vi "I2C_HostHandleIRQ_2.vi"(8 "error in":errorcluster, 10 "IRQ Number":i32, 11 "FPGA VI Reference In":T1) -> (0 "error out":errorcluster, 2 "Status":i16, 3 "FPGA VI Reference Out":T1)   [LabVIEW 2019]
doc: "Waits for the FPGA to update the specified IRQ. Once received it is acknowledged and the status is returned from the FPGA.\n\nVI Written By:\nPeter Fuller\nSenior Engineer\nplf Consulting, LLC"
uses:
  <vilib>/rvi/interface/nirviMethod/nirviMethod.xnode
  <vilib>/rvi/interface/nirviReadWriteControl/nirviReadWriteControl.xnode
  Controls/FPGA_Reference.ctl
  FPGA Bitfiles/LS_Durability_FPGA_9627.lvbitx
  <vilib>/rvi/interface/nirviMethod/StockFPGA_InlinedMethodWaitForSingleIRQ.vi
  <vilib>/FPGAPlugInAG/sbRIO-9627/niLvFpga_WaitOnIrq_sbRIO-9627.vi
  <vilib>/FPGAPlugInAG/sbRIO-9627/niLvFpga_AcknowledgeIrq_sbRIO-9627.vi
  <vilib>/rvi/errors/niLvFpgaMergeErrorWithErrorCode.vi
  <vilib>/rvi/errors/niLvFpgaAdjustHostInterfaceError.vi
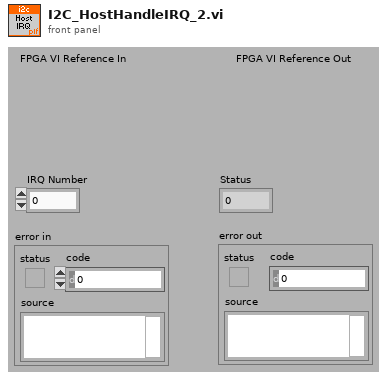
[diagram p1: front panel]
types:
  T1 = typedef "FPGA_Reference.ctl" = refnum<k20>
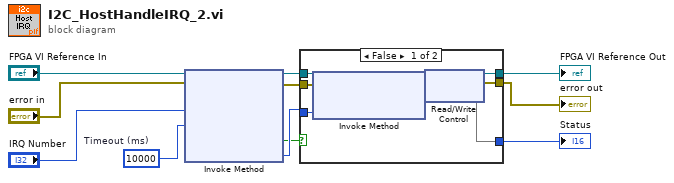
[diagram p0: block diagram]
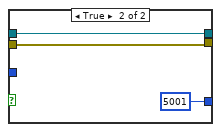
[diagram p2: hidden frame]
diagram:
  w7 = 10000  # Timeout (ms)
  n1 = xnode "Invoke Method"("FPGA VI Reference In"="FPGA VI Reference In", "error in"="error in", "IRQ Number(s)"="IRQ Number", "Timeout (ms)"=w7) -> ("FPGA VI Reference Out"=w4:T1, "error out"=w5:errorcluster, "Timed Out"=w6:bool, "IRQ(s) Asserted"=w9:i32)
  n2 = case shown="False" w6 {
    tunnel: w4 -> [w19 w21]
    tunnel: w5 -> [w18 w20]
    tunnel: w9 -> [w17 _]
    tunnel: [w14 w21] -> w1
    tunnel: [w13 w20] -> w2
    tunnel: [w12 i16 5001 ("Status")] -> w3
    frame False {
      n3 = xnode "Invoke Method"("FPGA VI Reference In"=w19, "error in"=w18, "IRQ Number(s)"=w17) -> ("FPGA VI Reference Out"=w16:T1, "error out"=w15:errorcluster)
      n4 = xnode "Read/Write Control"("FPGA VI Reference In"=w16, "error in"=w15) -> ("FPGA VI Reference Out"=w14:T1, "error out"=w13:errorcluster, "Status 2"=w12)
    }
    frame True {
    }
  }
  "Status" <- w3
  "error out" <- w2
  "FPGA VI Reference Out" <- w1
